vi "Logging File Header (SubVI).vi"(8 "Channel Name 2":string[](array[string])=["", "", "", "", "", "", "", "", "", "", "", "", "", "", "", "", "", "", "", "", "", "", "", "", "", "", "", "", "", "", "", ""], 9 "Channel Name":string[](array[string])=["", "", "", "", "", "", "", "", "", "", "", "", "", "", "", "", "", "", "", "", "", "", "", "", "", "", "", "", "", "", "", ""], 10 "error out":errorcluster, 11 "file (use dialog)":refnum<file>) -> (2 "error out 2":errorcluster, 3 "refnum out":refnum<file>)   [LabVIEW 2014]
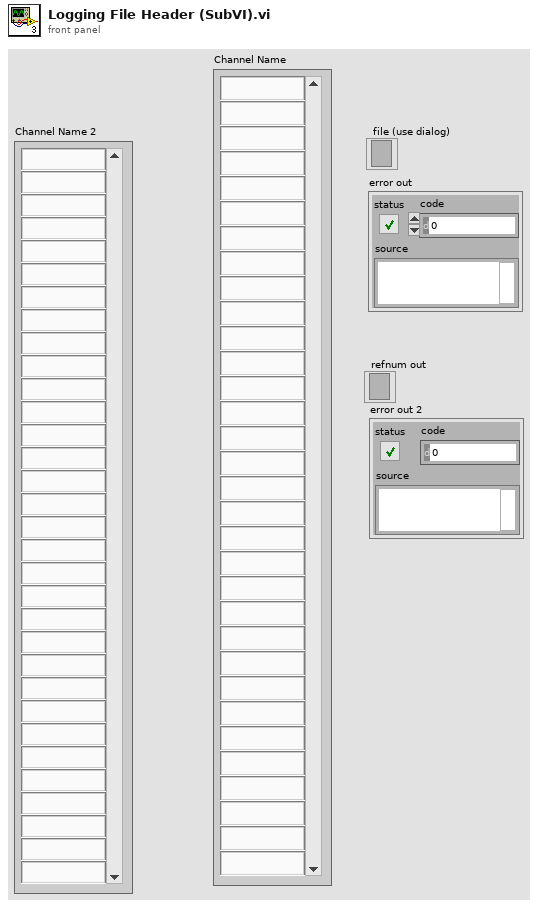
[diagram p1: front panel]
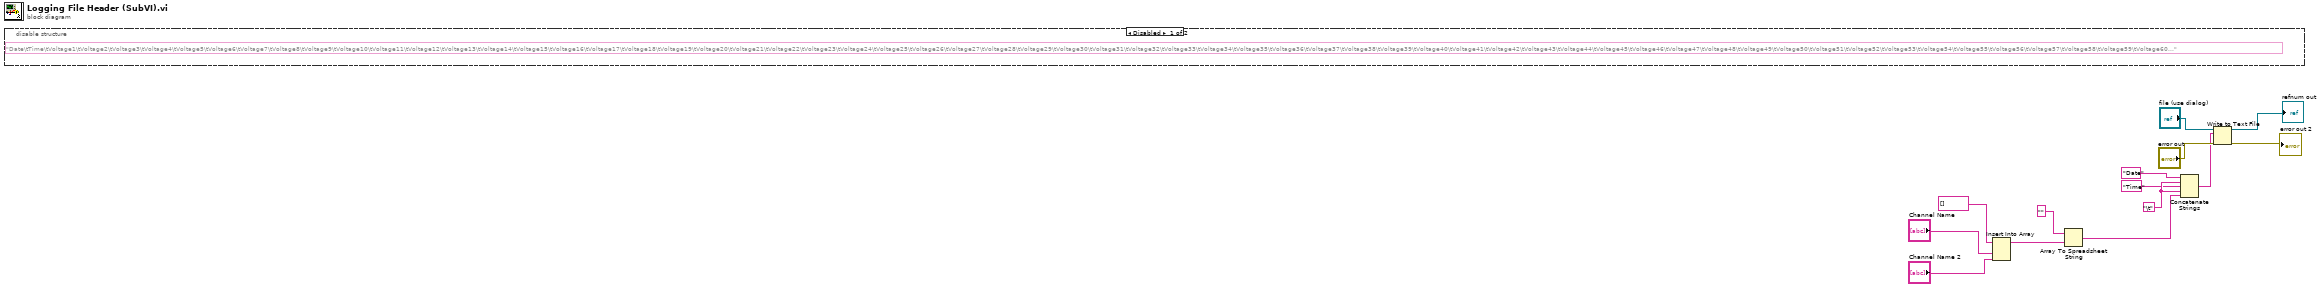
[diagram p0: block diagram]
diagram:
  w9 = "\t"
  n1 = disable-structure shown="Disabled" {
    frame Disabled {
      (unwired) "Date\tTime\tVoltage1\tVoltage2\tVoltage3\tVoltage4\tVoltage5\tVoltage6\tVoltage7\tVoltage8\tVoltage9\tVoltage10\tVoltage11\tVoltage12\tVoltage13\tVoltage14\tVoltage15\tVoltage16\tVoltage17\tVoltage18\tVoltage19\tVoltage20\tVoltage21\tVoltage22\tVoltage23\tVoltage24\tVoltage25\tVoltage26\tVoltage27\tVoltage28\tVoltage29\tVoltage30\tVoltage31\tVoltage32\tVoltage33\tVoltage34\tVoltage35\tVoltage36\tVoltage37\tVoltage38\tVoltage39\tVoltage40\tVoltage41\tVoltage42\tVoltage43\tVoltage44\tVoltage45\tVoltage46\tVoltage47\tVoltage48\tVoltage49\tVoltage50\tVoltage51\tVoltage52\tVoltage53\tVoltage54\tVoltage55\tVoltage56\tVoltage57\tVoltage58\tVoltage59\tVoltage60\tVoltage61\tVoltage62\tVoltage63\tVoltage64\r" ("text")
    }
    frame Enabled {
    }
  }
  n2 = Insert Into Array(array=string[] [], new element #1="Channel Name", new element #2="Channel Name 2") -> (w3:string[])  [unwired: 1 in]
  n3 = Array To Spreadsheet String(array=w3, 3:"" ("format string")) -> (spreadsheet string=w8:string)  [unwired: 1 in]
  n4 = Concatenate Strings("Date" ("string"), w9, "Time" ("string"), w9, w8) -> (w7:string)
  n5 = Write to Text File(file (use dialog)="file (use dialog)", text=w7, error in="error out") -> (refnum out=→"refnum out":refnum<file>, error out=→"error out 2":errorcluster)  [unwired: 1 in, 1 out]
